vi "Navigation_no s curve may 2 encoders.vi"() -> ()   [LabVIEW 2015]
uses:
  <vilib>/myRIO/Instrument Drivers/Onboard IO/PWM/typedefs/PWM Reference.ctl
  <vilib>/myRIO/Common/Instrument Driver Framework/Utilities/typedefs/myRIO Generic Hardware Reference.ctl
  <vilib>/myRIO/Common/Instrument Driver Framework/Utilities/typedefs/Hardware Version Enum.ctl
  <vilib>/myRIO/Common/Instrument Driver Framework/Utilities/typedefs/myRIO v1.0 Reference.ctl
  <vilib>/myRIO/Common/Instrument Driver Framework/Utilities/typedefs/Generic FPGA Reference.ctl
  <vilib>/myRIO/Common/Instrument Driver Framework/myRIO v1.0/PWM/typedefs/PWM Channels Enum.ctl
  <vilib>/myRIO/Instrument Drivers/Onboard IO/PWM/typedefs/PWM Configuration.ctl
  <vilib>/userdefined/High Color/nirio_resource_hc.ctl
  <vilib>/myRIO/Common/Instrument Driver Framework/myRIO v1.0/PWM/vis/myRIO v1.1 Open PWM.vi
  <vilib>/myRIO/Common/Instrument Driver Framework/Utilities/vis/Validate Channels.vi
  <vilib>/myRIO/Common/Instrument Driver Framework/myRIO v1.0/PWM/vis/myRIO v1.0 Reserve PWM.vi
  <vilib>/myRIO/Common/Instrument Driver Framework/myRIO v1.0/PWM/vis/myRIO v1.0 Build MUX Configuration PWM.vi
  <vilib>/myRIO/Common/Instrument Driver Framework/myRIO v1.0/Resource Manager/vis/myRIO v1.0 Reserve Channel List.vi
  <vilib>/myRIO/Common/Instrument Driver Framework/myRIO v1.0/Resource Manager/vis/myRIO v1.0 Create Configuration List.vi
  <vilib>/myRIO/Common/Instrument Driver Framework/myRIO v1.0/Resource Manager/vis/myRIO v1.0 Reserve Channel.vi
  <vilib>/myRIO/Common/Instrument Driver Framework/myRIO v1.0/Resource Manager/vis/myRIO v1.0 Unreserve Channel.vi
  <vilib>/myRIO/Common/Instrument Driver Framework/myRIO v1.0/Resource Manager/vis/myRIO v1.0 Build Mutex Name.vi
  <vilib>/FPGAPlugInAG/myRIO-1900/niLvFpga_Open_myRIO-1900.vi
  <vilib>/rvi/interface/common/dynamic/niFpgaDynamicAddResources.vi
  <vilib>/myRIO/Common/Instrument Driver Framework/Utilities/vis/FPGA Ref Manager.vi
  <vilib>/Utility/error.llb/Error Cluster From Error Code.vi
  <vilib>/myRIO/Common/Instrument Driver Framework/Utilities/vis/Ref Counter.vi
  <vilib>/rvi/errors/niLvFpgaAdjustHostInterfaceError.vi
  <vilib>/Utility/VariantDataType/GetNumericInfo.vi
  <vilib>/myRIO/Common/Instrument Driver Framework/myRIO v1.0/myRIO v1.1 Open.vi
  <vilib>/myRIO/Common/Instrument Driver Framework/Utilities/vis/IO Manager.vi
  <vilib>/myRIO/Common/Instrument Driver Framework/Utilities/vis/Configuration Manager.vi
  <vilib>/myRIO/Common/Instrument Driver Framework/myRIO v1.0/Resource Manager/vis/myRIO v1.0 Configure IO.vi
  <vilib>/myRIO/Common/Instrument Driver Framework/myRIO v1.0/myRIO v1.0 Close.vi
  <vilib>/myRIO/Common/Instrument Driver Framework/myRIO v1.0/PWM/vis/myRIO v1.0 Write PWM.vi
  <vilib>/addons/control/pid/pid.llb/PID (DBL).vi
  <vilib>/rvi/interface/nirviOpenFPGA/nirviOpenFPGA.xnode
  FPGA Bitfiles/NavigationProjec_FPGATarget2_FPGAMainNavigati_PWPHW8gwDxI.lvbitx
  <vilib>/rvi/interface/nirviReadWriteControl/nirviReadWriteControl.xnode
  <vilib>/myRIO/Instrument Drivers/Onboard IO/PWM/vis/myRIO PWM Open.xnode
  <vilib>/myRIO/Instrument Drivers/Onboard IO/PWM/PWM.lvlib
  <vilib>/myRIO/Instrument Drivers/Utilities/Utilities.lvlib
  NiFpgaLv.dll
  <vilib>/rvi/interface/Simulation/niFpgaSimulationCallBeginRW.vi
  <vilib>/addons/control/pid/NI_PID_pid.lvlib
panel:
  out "percent to goal":dbl
  out "x goal current":dbl=8.0
  out "big red button":i16
  out "y1ahead":dbl
  out "angle error":dbl
  out "y desired":dbl
  out "slope desired":dbl
  out "orientation theta desired":dbl
  out "current angle":dbl
  out "current y":dbl
  out "current x":dbl
  out "mining angle":dbl
  out "mining y":dbl
  out "mining x":dbl
  out "mining location":dbl=1.0
  out "distance to goal":dbl
  out "loc_y":dbl
  out "loc_x":dbl
  out "loc_theta":dbl
  in  "motor killswitch":bool=TRUE
  in  "set start position":bool
  in  "dumping complete":bool
  in  "digging complete?":bool
  in  "position good?":bool
  in  "state":dbl
  in  "x goal":dbl=8.0
  in  "Encoder Reset":bool
  out "scale":dbl=1.0
  out "reset x y 2":dbl
  out "stop motors":dbl
  out "encoder stop switch":dbl=1.0
  out "left wheels actual pwm":dbl
  out "right wheels actual pwm":dbl
  out "desired pwm right":dbl
  out "desired pwm left":dbl
  out "left setpoint":dbl
  out "right setpoint":dbl
  in  "PID Settings":enum32{"Right PID PWM", "Left PID PWM"}(tab)
  in  "output range right":cluster{"output high":dbl, "output low":dbl}={"output high"=0.13333, "output low"=-0.13333} {"output low" format="%.6f"; "output high" format="%.5f"}
  in  "PID gains right":T1={"proportional gain (Kc)"=0.002, "integral time (Ti, min)"=7e-07, "derivative time (Td, min)"=0.0} {"derivative time (Td, min)" format="%.8f"; "integral time (Ti, min)" format="%.8f"; "proportional gain (Kc)" format="%.8f"}
  out "dt out (s) right":dbl format="%.3f"
  out "PID feedback Right":dbl
  out "Elapsed Time (s) Right":dbl caption="Elapsed Time (s)"
  in  "pid reset right":bool
  in  "output range left":cluster{"output high":dbl, "output low":dbl}={"output high"=0.13333, "output low"=-0.13333} {"output low" format="%.6f"; "output high" format="%.5f"}
  in  "PID gains left":T1={"proportional gain (Kc)"=0.002, "integral time (Ti, min)"=7e-07, "derivative time (Td, min)"=0.0} {"derivative time (Td, min)" format="%.8f"; "integral time (Ti, min)" format="%.8f"; "proportional gain (Kc)" format="%.8f"}
  out "dt out (s) left":dbl format="%.3f"
  out "PID feedback Left":dbl
  out "Elapsed Time (s) Left":dbl caption="Elapsed Time (s)"
  in  "pid reset left":bool
  out "start angle":dbl=1.0
  out "start x":dbl=1.0
  out "start y":dbl
  in  "stuff that i dont want to mess with right now":T2(tab)
  out "RM Linear Velocity (rot/s)":dbl
  out "RR Rot Velocity (rot/s)":dbl
  out "LR Rot Velocity (rot/s)":dbl
  out "LM Rot Velocity (rot/s)":dbl
  out "LF Rot Velocity (rot/s)":dbl
  out "RF Linear Velocity (rot/s)":dbl
  out "Tick Count(mSec) 2":u32 caption="Tick Count(mSec)"
  out "y traveled 2":dbl
  out "x traveled 2":dbl
  out "y position 2":dbl
  out "x position 2":dbl
  out "y dot 2":dbl
  out "distance traveled 2":dbl
  out "psi dot 2":dbl
  out "x dot 2":dbl
  out ".not. x? 2":bool
  out ".not. x? 3":bool
  out "goal reached":bool=TRUE
  out "avg ENC.B":dbl
  out "avg ENC.A":dbl
  out "ENC.B_c.CNTR":i32
  out "ENC.B_b.CNTR":i32
  out "ENC.B_a.CNTR":i32
  out "ENC.A_c.CNTR":i32
  out "ENC.A_b.CNTR":i32
  out "ENC.A_a.CNTR":i32
  out "stage set point parameters":T3(tab)
  in  "x straight 1 end":dbl=2.0
  in  "ypstart straight 1":dbl
  in  "ystart":dbl=1.0
  in  "yend straight 1":dbl=2.0
  in  "ypend straight 1":dbl
  out "a":dbl
  out "b":dbl
  out "c":dbl
  out "d":dbl
  out "x turn end":dbl=7.0
  out "x straight 2 end":dbl=10.0
  in  "mining y 1":dbl=2.0
  in  "mining angle 1":dbl
  in  "mining x 1":dbl=-8.0
  in  "mining angle -1":dbl
  in  "mining y -1":dbl=4.0
  in  "mining x -1":dbl=-8.0
  out "left pwm":dbl(graph)
  out "right pwm":dbl(graph)
  out "SYS.SELECTA":u8 format="%08b"
  in  "R Min Linear Velocity (ft/s)":dbl=-2.0 format="%#_13g"
  in  "R Max Linear Velocity (ft/s)":dbl=2.0 format="%#_13g"
  in  "L Min Linear Velocity (ft/s)":dbl=-2.0 format="%#_13g"
  in  "L Max Linear Velocity (ft/s)":dbl=2.0 format="%#_13g"
  out "Current Rot Velocity (rot/s)":T4(graph)
  # "Position Information"
  # "move cases along"
  # "end state 0\ngo to state 1"
  # "end state 1\ngo to state 2"
  # "end state 2\ngo to state 3"
  # "end state 3\ngo to state 4"
  # "end state 4\ngo to state 0"
  # "same thing, redundant \nbut can be changed to \nsomething useful later"
  # "this must be true to \ninitialize the routine"
  # "go through the 3\n movement cases"
  # "go through the 3\n movement cases"
  # "Stop Flags \n1=go \n0=stop"
  # "PWM Setpoint"
  # "Initial condtions"
  # "Encoder Values"
  # "Motor Control Parameters"
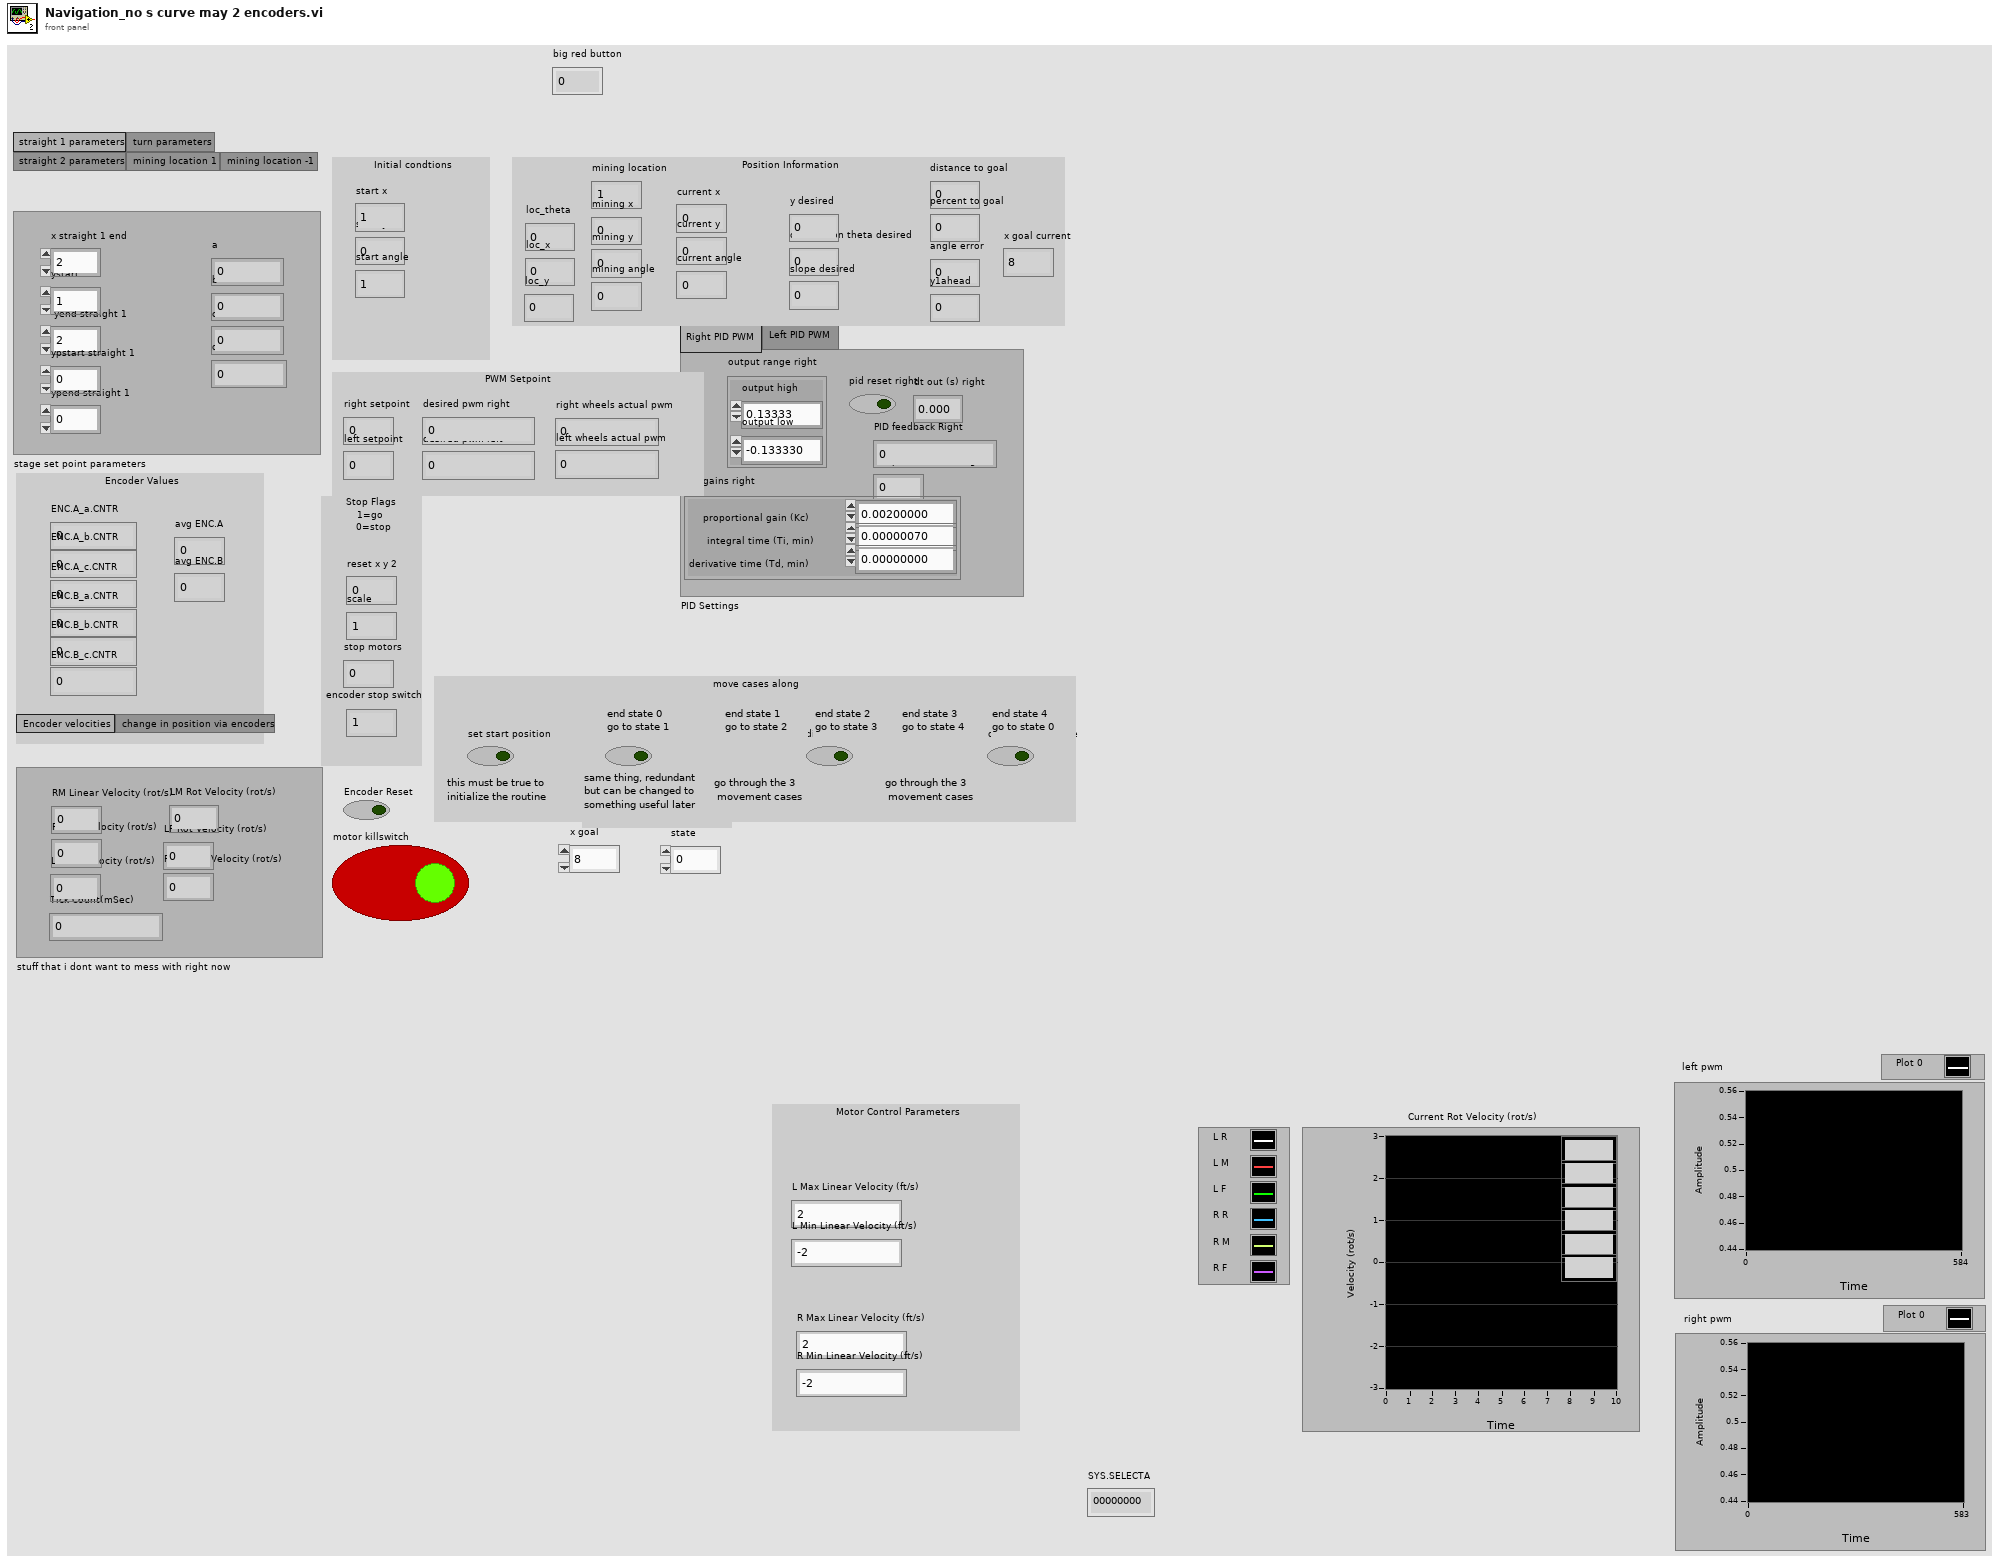
[diagram p1: front panel]
types:
  T1 = cluster{"proportional gain (Kc)":dbl, "integral time (Ti, min)":dbl, "derivative time (Td, min)":dbl}
  T2 = enum32{"Encoder velocities", "change in position via encoders"}
  T3 = enum32{"straight 1 parameters", "turn parameters", "straight 2 parameters", "mining location 1", "mining location -1"}
  T4 = cluster{"Rotational Velocity (RPS)":dbl, "Rotational Velocity (RPS)":dbl, "Rotational Velocity (RPS)":dbl, "Rotational Velocity (RPS)":dbl, "Rotational Velocity (RPS)":dbl, "Rotational Velocity (RPS)":dbl}
  T5 = typedef "nirio_resource_hc.ctl" = tag
  T6 = typedef "Hardware Version Enum.ctl" = enum16{"Unknown", "myRIO-1900", "myRIO-1950", "roboRIO"}
  T7 = typedef "PWM.lvlib/PWM Reference.ctl" = cluster{"myRIO Reference":T8, "PWM Channels Enum":T11, "PWM Configuration":T12}
  T8 = typedef "myRIO Generic Hardware Reference.ctl" = cluster{"myRIO Model":T6, "myRIO Hardware Reference":T9}
  T9 = typedef "myRIO v1.0 Reference.ctl" = cluster{"Generic FPGA Reference":T10, "Allow multiple opens":bool}
  T10 = typedef "Generic FPGA Reference.ctl" = refnum<k20>
  T11 = typedef "PWM Channels Enum.ctl" = enum16{"Not Connected", "C/PWM0", "C/PWM1", "A/PWM0", "A/PWM1", "A/PWM2", "B/PWM0", "B/PWM1", "B/PWM2", "PWM/PWM0", "PWM/PWM1", "PWM/PWM2", "PWM/PWM3", "PWM/PWM4", "PWM/PWM5", "PWM/PWM6", "PWM/PWM7", "PWM/PWM8", "PWM/PWM9"}
  T12 = typedef "PWM.lvlib/PWM Configuration.ctl" = cluster{"Frequency":dbl, "Duty Cycle":dbl}
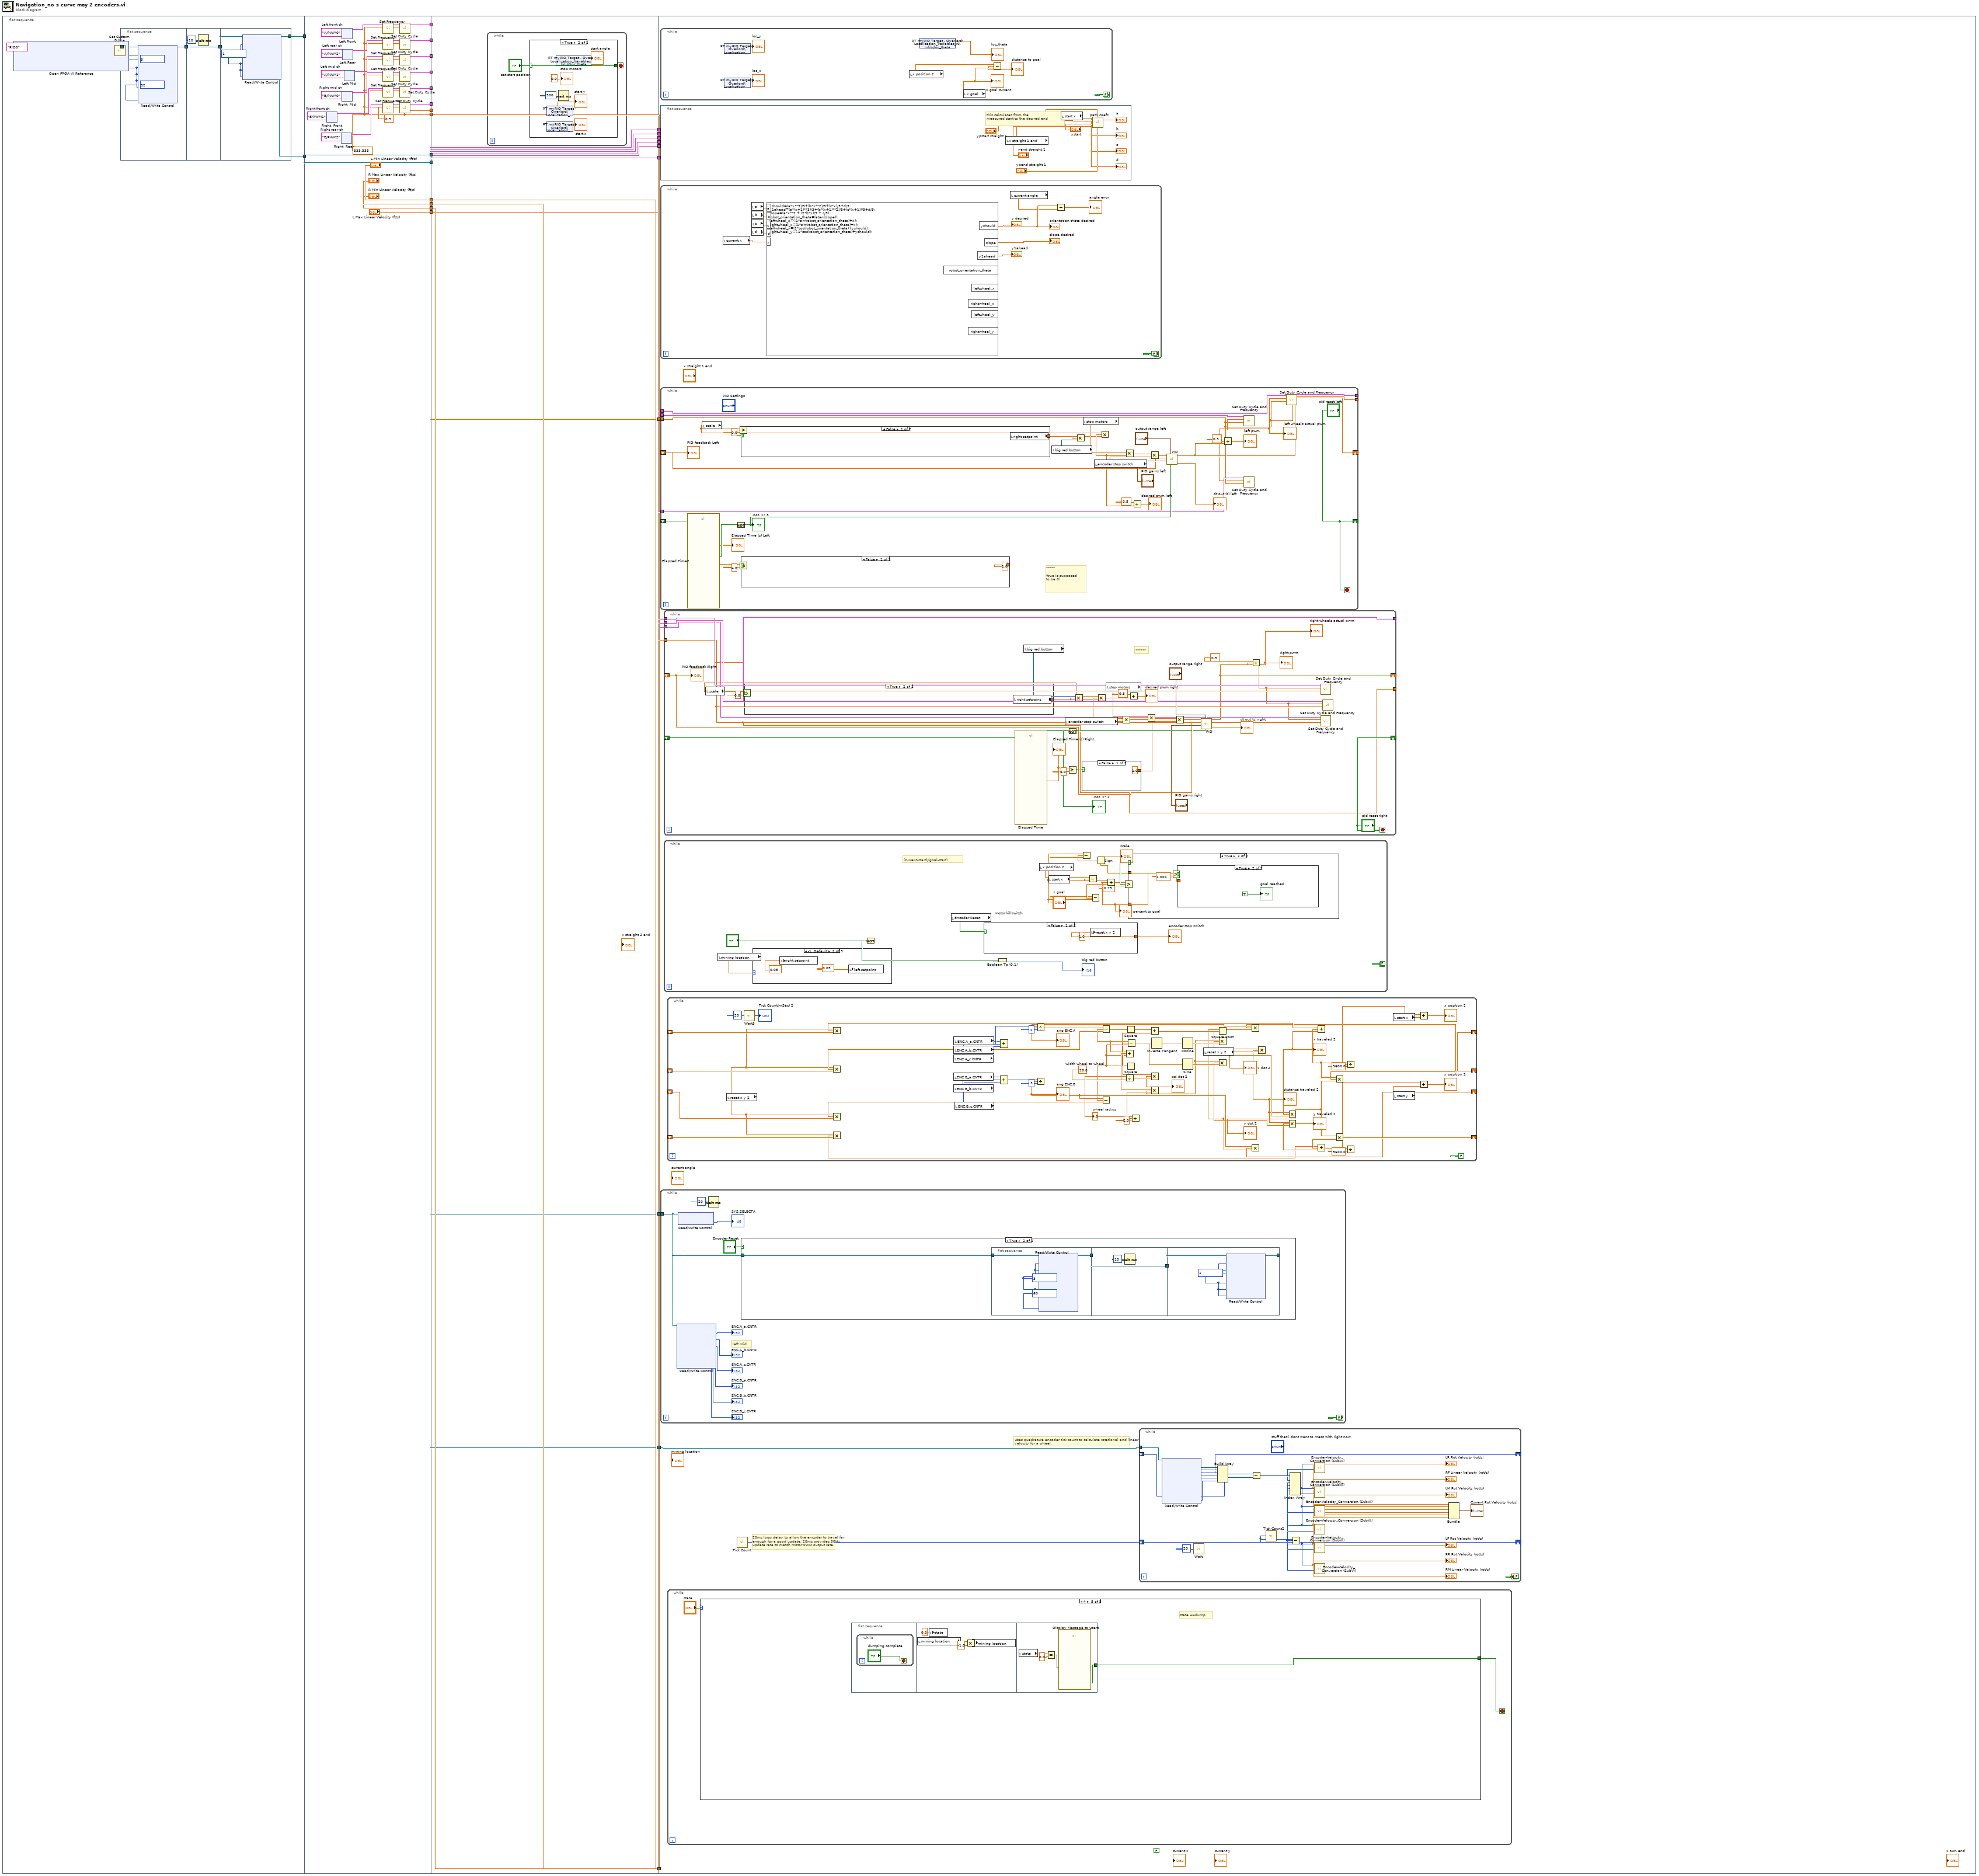
[diagram p0: block diagram]
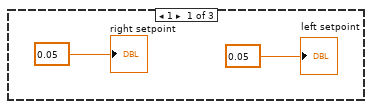
[diagram p3: hidden frame]
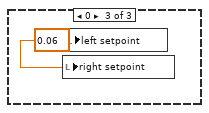
[diagram p4: hidden frame]
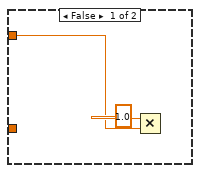
[diagram p5: hidden frame]
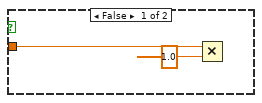
[diagram p6: hidden frame]
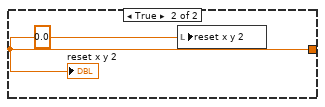
[diagram p7: hidden frame]
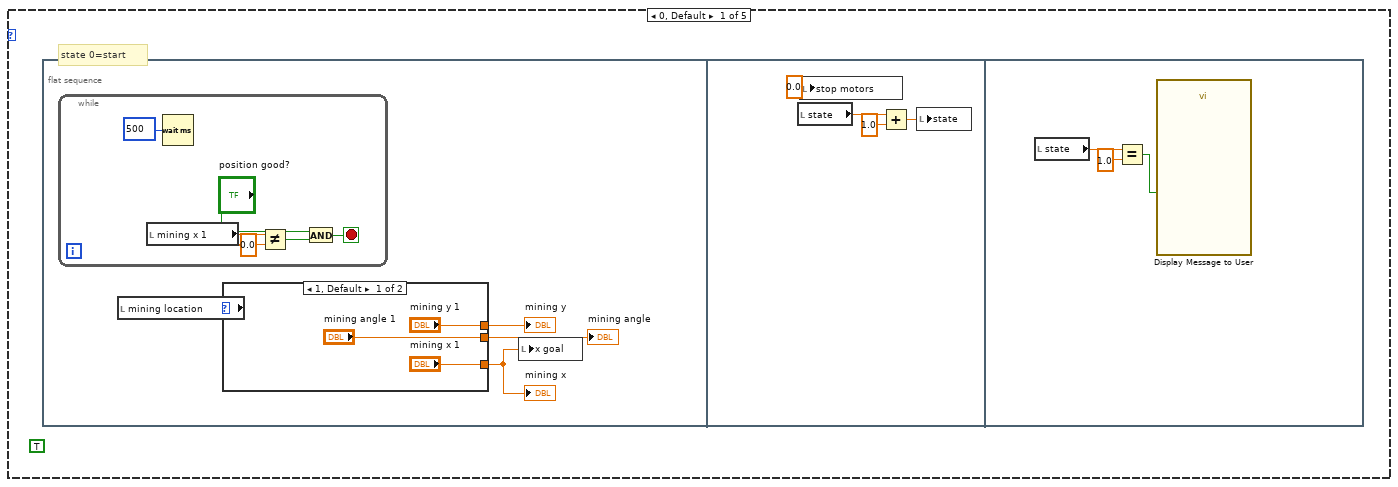
[diagram p8: hidden frame]
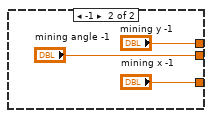
[diagram p9: hidden frame]
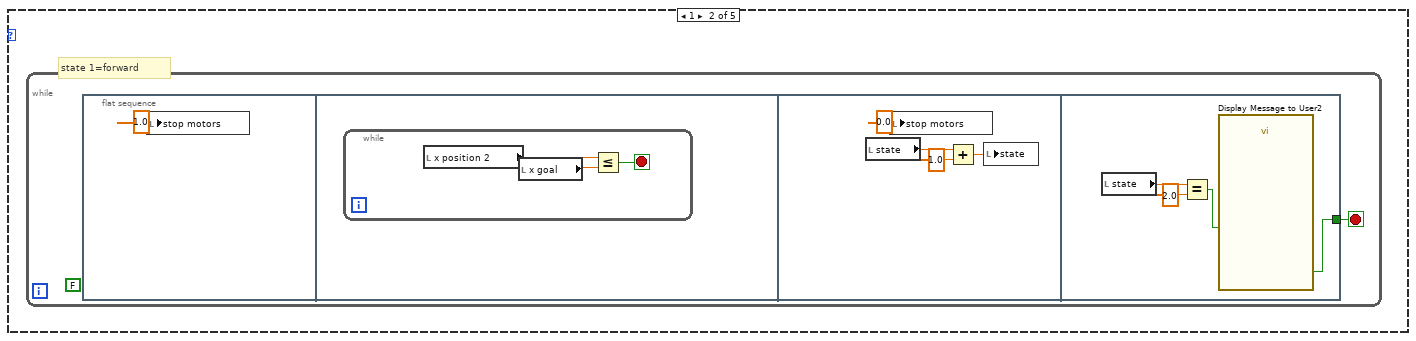
[diagram p10: hidden frame]
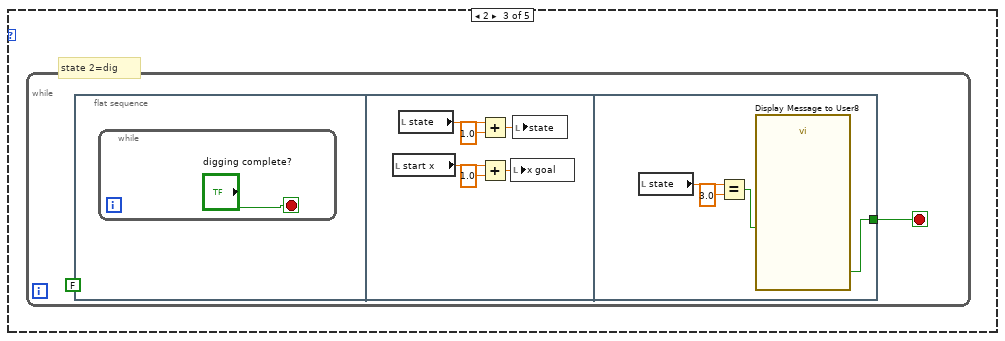
[diagram p11: hidden frame]
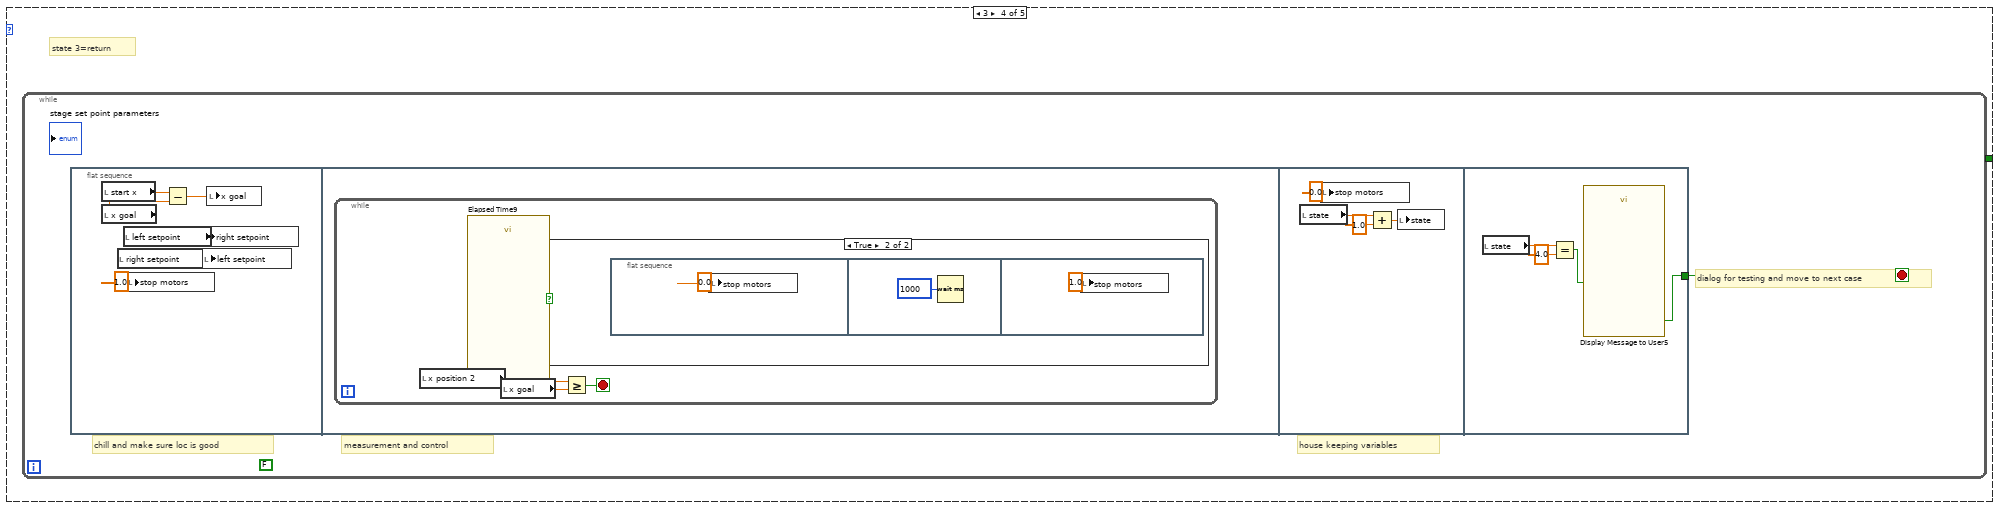
[diagram p12: hidden frame]
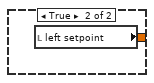
[diagram p14: hidden frame]
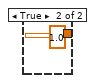
[diagram p15: hidden frame]
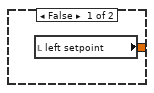
[diagram p16: hidden frame]
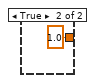
[diagram p17: hidden frame]
diagram:
  n1 = flat-sequence {
    tunnel: [w33] -> w30
    tunnel: [w33] -> w29
    tunnel: [w46] -> w28
    tunnel: [w61] -> w26
    tunnel: [w57] -> w24
    tunnel: [w56] -> w22
    tunnel: [w55] -> w20
    tunnel: [w54] -> w18
    tunnel: [w53] -> w16
    tunnel: ["L Max Linear Velocity (ft/s)"] -> w14
    tunnel: ["L Min Linear Velocity (ft/s)"] -> w12
    tunnel: ["R Max Linear Velocity (ft/s)"] -> w10
    tunnel: ["R Min Linear Velocity (ft/s)"] -> w8
    tunnel: [w48] -> w6
    tunnel: w30 -> [w47]
    tunnel: [w47] -> w4
    tunnel: w29 -> [w48]
    tunnel: [w46] -> w2
    tunnel: w28 -> [w187]
    tunnel: [w187] -> w27
    tunnel: w26 -> [w186]
    tunnel: [w186] -> w25
    tunnel: w24 -> [w185]
    tunnel: [w185] -> w23
    tunnel: w22 -> [w184]
    tunnel: [w184] -> w21
    tunnel: w20 -> [w183]
    tunnel: [w183] -> w19
    tunnel: w18 -> [w182]
    tunnel: [w182] -> w17
    tunnel: w16 -> [w181]
    tunnel: [w181] -> w15
    tunnel: w14 -> [w180]
    tunnel: [w180] -> w13
    tunnel: w12 -> [w179]
    tunnel: [w179] -> w11
    tunnel: w10 -> [w178]
    tunnel: [w178] -> w9
    tunnel: w8 -> [w177]
    tunnel: [w177] -> w7
    tunnel: w6 -> [w176]
    tunnel: [w176] -> w5
    tunnel: w4 -> [w175]
    tunnel: [w175] -> w3
    tunnel: w2 -> [w174]
    tunnel: [w174] -> w1
    tunnel: w27 -> [_]
    tunnel: w25 -> [w196]
    tunnel: w23 -> [w202]
    tunnel: w21 -> [w199]
    tunnel: w19 -> [w198]
    tunnel: w17 -> [w197]
    tunnel: w15 -> [w201]
    tunnel: w13 -> [_]
    tunnel: w11 -> [_]
    tunnel: w9 -> [_]
    tunnel: w7 -> [_]
    tunnel: w5 -> [w204]
    tunnel: w3 -> [w203]
    tunnel: w1 -> [w200]
    frame #0 {
      n2 = xnode "Open FPGA VI Reference"("resource name"=tag "RIO0") -> ("FPGA VI Reference Out"=w32:refnum<k20>)  [unwired: 1 in, 1 out]
      n3 = call <vilib>:"Set Custom Bitfile.vi"("Custom FPGA Reference In"=w32) -> ("Custom FPGA Reference Out"=w34:refnum<k20>)  [unwired: 9 in, 1 out]
      n4 = flat-sequence {
        tunnel: w34 -> [w39]
        tunnel: [w37] -> w36
        tunnel: w36 -> [w41]
        tunnel: [w41] -> w35
        tunnel: w35 -> [w44]
        tunnel: [w43] -> w33
        frame #0 {
          w38 = u8 32 ("SYS.SELECTA")
          w40 = u8 3 ("ENC.B_c.CNFG")
          n5 = xnode "Read/Write Control"("FPGA VI Reference In"=w39, "ENC.A_a.CNFG"=w40, "ENC.A_b.CNFG"=w40, "ENC.A_c.CNFG"=w40, "ENC.B_a.CNFG"=w40, "ENC.B_b.CNFG"=w40, "ENC.B_c.CNFG"=w40, "SYS.SELECTA"=w38, "SYS.SELECTB"=w38) -> ("FPGA VI Reference Out"=w37:refnum<k20>)  [unwired: 1 in, 1 out]
        }
        frame #1 {
          n6 = Wait (ms)(milliseconds to wait=u32 10) -> ()  [unwired: 1 out]
        }
        frame #2 {
          w45 = u8 1 ("ENC.B_c.CNFG")
          n7 = xnode "Read/Write Control"("FPGA VI Reference In"=w44, "ENC.A_a.CNFG"=w45, "ENC.A_b.CNFG"=w45, "ENC.A_c.CNFG"=w45, "ENC.B_a.CNFG"=w45, "ENC.B_b.CNFG"=w45, "ENC.B_c.CNFG"=w45) -> ("FPGA VI Reference Out"=w43:refnum<k20>)  [unwired: 1 in, 1 out]
        }
      }
    }
    frame #1 {
      w58 = 0.5 ("Duty Cycle")
      w46 = 333.333 ("Frequency [Hz]")
      w72 = tag "B/PWM2"  # Right rear ch
      w73 = tag "B/PWM0"  # Right mid ch
      w74 = tag "B/PWM1"  # Right front ch
      w75 = tag "A/PWM2"  # Left rear ch
      w76 = tag "A/PWM1"  # Left mid ch
      w77 = tag "A/PWM0"  # Left front ch
      n8 = xnode "Right  Front"("Channel Name"=w74) -> ("PWM Ref Out"=w68:T7)  [unwired: 2 in, 1 out]
      n9 = xnode "Right  Rear"("Channel Name"=w72) -> ("PWM Ref Out"=w66:T7)  [unwired: 2 in, 1 out]
      n10 = xnode "Left Front"("Channel Name"=w77) -> ("PWM Ref Out"=w71:T7)  [unwired: 2 in, 1 out]
      n11 = xnode "Right  Mid"("Channel Name"=w73) -> ("PWM Ref Out"=w67:T7)  [unwired: 2 in, 1 out]
      n12 = xnode "Left Rear"("Channel Name"=w75) -> ("PWM Ref Out"=w69:T7)  [unwired: 2 in, 1 out]
      n13 = xnode "Left Mid"("Channel Name"=w76) -> ("PWM Ref Out"=w70:T7)  [unwired: 2 in, 1 out]
      n14 = call <vilib>:"Set Frequency.vi"("Frequency [Hz]"=w46, "PWM Ref In"=w71) -> ("PWM Ref Out"=w65:T7)  [unwired: 7 in, 1 out]
      n15 = call <vilib>:"Set Frequency.vi"("Frequency [Hz]"=w46, "PWM Ref In"=w69) -> ("PWM Ref Out"=w60:T7)  [unwired: 7 in, 1 out]
      n16 = call <vilib>:"Set Frequency.vi"("Frequency [Hz]"=w46, "PWM Ref In"=w70) -> ("PWM Ref Out"=w59:T7)  [unwired: 7 in, 1 out]
      n17 = call <vilib>:"Set Frequency.vi"("Frequency [Hz]"=w46, "PWM Ref In"=w67) -> ("PWM Ref Out"=w63:T7)  [unwired: 7 in, 1 out]
      n18 = call <vilib>:"Set Frequency.vi"("Frequency [Hz]"=w46, "PWM Ref In"=w68) -> ("PWM Ref Out"=w62:T7)  [unwired: 7 in, 1 out]
      n19 = call <vilib>:"Set Frequency.vi"("Frequency [Hz]"=w46, "PWM Ref In"=w66) -> ("PWM Ref Out"=w64:T7)  [unwired: 7 in, 1 out]
      n20 = call <vilib>:"Set Duty Cycle.vi"("Duty Cycle"=w58, "PWM Ref In"=w65) -> ("PWM Ref Out"=w53:T7)  [unwired: 7 in, 1 out]
      n21 = call <vilib>:"Set Duty Cycle.vi"("Duty Cycle"=w58, "PWM Ref In"=w60) -> ("PWM Ref Out"=w61:T7)  [unwired: 7 in, 1 out]
      n22 = call <vilib>:"Set Duty Cycle.vi"("Duty Cycle"=w58, "PWM Ref In"=w59) -> ("PWM Ref Out"=w54:T7)  [unwired: 7 in, 1 out]
      n23 = call <vilib>:"Set Duty Cycle.vi"("Duty Cycle"=w58, "PWM Ref In"=w63) -> ("PWM Ref Out"=w56:T7)  [unwired: 7 in, 1 out]
      n24 = call <vilib>:"Set Duty Cycle.vi"("Duty Cycle"=w58, "PWM Ref In"=w62) -> ("PWM Ref Out"=w57:T7)  [unwired: 7 in, 1 out]
      n25 = call <vilib>:"Set Duty Cycle.vi"("Duty Cycle"=w58, "PWM Ref In"=w64) -> ("PWM Ref Out"=w55:T7)  [unwired: 7 in, 1 out]
    }
    frame #2 {
      n26 = while {
        stop <- w188 stop-if-true
        n27 = case shown="True" "set start position" {
          selector: "set start position" -> [_ w195]
          tunnel: [_ w195] -> w188
          frame False {
          }
          frame True {
            n28 = shared-variable "RT myRIO Target - Overlord\\Localization_Variables_r0.lvlib\\loc_y"() -> (→"start y":dbl)  [unwired: 1 in, 1 out]
            n29 = shared-variable "RT myRIO Target - Overlord\\Localization_Variables_r0.lvlib\\loc_x"() -> (→"start x":dbl)  [unwired: 1 in, 1 out]
            n30 = shared-variable "RT myRIO Target - Overlord\\Localization_Variables_r0.lvlib\\loc_theta"() -> (→"start angle":dbl)  [unwired: 1 in, 1 out]
            n31 = Wait (ms)(milliseconds to wait=u32 500) -> ()  [unwired: 1 out]
            "stop motors" <- 0.0 ("stop motors")
          }
        }
      }
    }
    frame #3 {
      (unwired) FALSE
      # "Uses quadrature encoder tick count to calculate rotational and linear velocity for a wheel."
      # "20ms loop delay to allow the encoder to travel far enough for a good update. 20ms provides 50Hz update rate to match motor PWM output rate."
      n32 = while {
        stop <- FALSE stop-if-true
        n33 = shared-variable "RT myRIO Target - Overlord\\Localization_Variables_r0.lvlib\\loc_y"() -> (→"loc_y":dbl)  [unwired: 1 in, 1 out]
        n34 = shared-variable "RT myRIO Target - Overlord\\Localization_Variables_r0.lvlib\\loc_x"() -> (→"loc_x":dbl)  [unwired: 1 in, 1 out]
        n35 = local read "x position 2"() -> (w343:dbl)
        n36 = shared-variable "RT myRIO Target - Overlord\\Localization_Variables_r0.lvlib\\loc_theta"() -> (→"loc_theta":dbl)  [unwired: 1 in, 1 out]
        n37 = local read "x goal"() -> (w346:dbl)
        "x goal current" <- w346
        n38 = Subtract(x=w343, y=w346) -> (x-y=→"distance to goal":dbl)
      }
      n39 = flat-sequence {
        frame #0 {
          # "this calculates from the \nmeasured start to the desired end"
          n40 = local read "x straight 1 end"() -> (w251:dbl)
          n41 = local read "start x"() -> (w252:dbl)
          n42 = call "path coefs.vi"("ypend"="ypend straight 1", "ypstart"="ypstart straight 1", "yend"="yend straight 1", "ystart"="ystart", "xend"=w251, "xstart"=w252) -> ("d"=→"d":dbl, "c"=→"c":dbl, "b"=→"b":dbl, "a"=→"a":dbl)  [unwired: 2 in]
        }
      }
      n43 = while {
        stop <- FALSE stop-if-true
        n44 = local read "current x"() -> (w245:dbl)
        n45 = local read "a"() -> (w249:dbl)
        n46 = local read "b"() -> (w248:dbl)
        n47 = local read "d"() -> (w246:dbl)
        n48 = local read "c"() -> (w247:dbl)
        n49 = formula code="yshould=(a*x**3)/3+(b*x**2)/3+(c*x)/3+d/3;\ny1ahead=(a*(x+1)**3)/3+(b*(x+1)**2)/3+(c*(x+1))/3+d/3;\nslope=(a*x**2 + (2*b*x)/3 + c/3);\nrobot_orientation_theta=(atan(slope));\nleftwheel_x=(-1*sin(robot_orientation_theta)+x);\nrightwheel_x=(1*sin(robot_orientation_theta)+x);\nleftwheel_y=(1*cos(robot_orientation_theta)+yshould);\nrightwheel_y=(-1*cos(robot_orientation_theta)+yshould);"("a"=w249, "b"=w248, "c"=w247, "d"=w246, "x"=w245) -> ("yshould"=→"y desired":dbl, "slope"=→"slope desired":dbl, "robot_orientation_theta"=w242:dbl, "y1ahead"=→"y1ahead":dbl)  [unwired: 4 out]
        "orientation theta desired" <- w242
        n50 = local read "current angle"() -> (w241:dbl)
        n51 = Subtract(x=w242, y=w241) -> (x-y=→"angle error":dbl)
      }
      n52 = while {
        tunnel: w201 -> [w380]
        tunnel: [w381] -> _
        tunnel: w200 -> [w368]
        shift-right: [w367] -> _
        shift-left: _ -> [w376]
        shift-right: ["pid reset left"] -> _
        shift-left: _ -> [w362]
        tunnel: [w368] -> _
        tunnel: w197 -> [w370]
        tunnel: w196 -> [w369]
        stop <- "pid reset left" stop-if-true
        # "*****\n\n(true is supposed\nto be 0)"
        n53 = call "Elapsed Time2"("Reset"=w362) -> ("Elapsed Time (s)"=w361:dbl, "Time has Elapsed"=w363:bool)  [unwired: 11 in, 6 out]
        "Elapsed Time (s) Left" <- w361
        n54 = local read "scale"() -> (w353:dbl)
        n55 = Not(x=w363) -> (.not. x?=w375:bool)
        ".not. x? 3" <- w375
        n56 = Greater?(x=w353, y=0.0) -> (0:w356:bool)
        n57 = Greater Or Equal?(x=w361, y=4.0) -> (x >= y?=w359:bool)
        n58 = case shown="False" w356 {
          tunnel: [w382 w383] -> w366
          frame False {
            n59 = local read "right setpoint"() -> (w382:dbl)
          }
          frame True {
            n60 = local read "left setpoint"() -> (w383:dbl)
          }
        }
        n61 = case shown="False" w359 {
          tunnel: [1.0 1.0] -> _
          frame False {
          }
          frame True {
          }
        }
        n62 = local read "big red button"() -> (w350:i16)
        n63 = Multiply(x=w366, y=w350) -> (x*y=w351:dbl)
        n64 = local read "stop motors"() -> (w371:dbl)
        n65 = local read "encoder stop switch"() -> (w364:dbl)
        n66 = Multiply(x=w353, y=w351) -> (x*y=w354:dbl)
        n67 = Multiply(x=w371, y=w354) -> (x*y=w365:dbl)
        n68 = Add(x=0.5, y=w354) -> (x+y=→"desired pwm left":dbl)
        n69 = Multiply(x=w365, y=w364) -> (x*y=w352:dbl)
        n70 = call-poly <vilib>:"PID.vi"("reinitialize? (F)"=w375, "output range"="output range left", "PID gains"="PID gains left", "process variable"=w376, "setpoint"=w352) -> ("dt out (s)"=→"dt out (s) left":dbl, "output"=w367:dbl)  [unwired: 5 in]
        n71 = Add(x=0.5, y=w367) -> (x+y=w357:dbl)
        "left wheels actual pwm" <- w357
        "left pwm" <- w357
        n72 = call <vilib>:"Set Duty Cycle and Frequency.vi"("Frequency [Hz]"=w368, "Duty Cycle"=w357, "PWM Ref In"=w369) -> ()  [unwired: 6 in, 2 out]
        n73 = call <vilib>:"Set Duty Cycle and Frequency.vi"("Frequency [Hz]"=w368, "Duty Cycle"=w357, "PWM Ref In"=w370) -> ()  [unwired: 6 in, 2 out]
        n74 = call <vilib>:"Set Duty Cycle and Frequency.vi"("Frequency [Hz]"=w368, "Duty Cycle"=w357, "PWM Ref In"=w380) -> ("PWM Ref Out"=w381:T7)  [unwired: 6 in, 1 out]
        "PID feedback Left" <- w376
      }
      n75 = while {
        tunnel: w204 -> [w486]
        stop <- FALSE stop-if-true
        # "left mid"
        n76 = xnode "Read/Write Control"("FPGA VI Reference In"=w486) -> ("ENC.A_a.CNTR"=→"ENC.A_a.CNTR":u32, "ENC.A_b.CNTR"=→"ENC.A_b.CNTR":u32, "ENC.A_c.CNTR"=→"ENC.A_c.CNTR":u32, "ENC.B_a.CNTR"=→"ENC.B_a.CNTR":u32, "ENC.B_b.CNTR"=→"ENC.B_b.CNTR":u32, "ENC.B_c.CNTR"=→"ENC.B_c.CNTR":u32)  [unwired: 1 in, 2 out]
        n77 = xnode "Read/Write Control"("FPGA VI Reference In"=w486) -> ("SYS.SELECTA"=→"SYS.SELECTA":u8)  [unwired: 1 in, 2 out]
        n78 = Wait (ms)(milliseconds to wait=u32 20) -> ()  [unwired: 1 out]
        n79 = case shown="True" "Encoder Reset" {
          tunnel: w486 -> [_ w497]
          frame False {
          }
          frame True {
            n80 = flat-sequence {
              tunnel: w497 -> [w502]
              tunnel: [w500] -> w499
              tunnel: w499 -> [w504]
              tunnel: [w504] -> w498
              tunnel: w498 -> [w507]
              tunnel: [w506] -> _
              frame #0 {
                w501 = u8 60 ("SYS.SELECTA")
                w503 = u8 3 ("ENC.B_c.CNFG")
                n81 = xnode "Read/Write Control"("FPGA VI Reference In"=w502, "ENC.A_a.CNFG"=w503, "ENC.A_b.CNFG"=w503, "ENC.A_c.CNFG"=w503, "ENC.B_a.CNFG"=w503, "ENC.B_b.CNFG"=w503, "ENC.B_c.CNFG"=w503, "SYS.SELECTA"=w501, "SYS.SELECTB"=w501) -> ("FPGA VI Reference Out"=w500:refnum<k20>)  [unwired: 1 in, 1 out]
              }
              frame #1 {
                n82 = Wait (ms)(milliseconds to wait=u32 10) -> ()  [unwired: 1 out]
              }
              frame #2 {
                w508 = u8 1 ("ENC.B_c.CNFG")
                n83 = xnode "Read/Write Control"("FPGA VI Reference In"=w507, "ENC.A_a.CNFG"=w508, "ENC.A_b.CNFG"=w508, "ENC.A_c.CNFG"=w508, "ENC.B_a.CNFG"=w508, "ENC.B_b.CNFG"=w508, "ENC.B_c.CNFG"=w508) -> ("FPGA VI Reference Out"=w506:refnum<k20>)  [unwired: 1 in, 1 out]
              }
            }
          }
        }
      }
      n84 = while {
        tunnel: w202 -> [w480]
        tunnel: [w481] -> _
        tunnel: [w469] -> _
        shift-right: [w468] -> _
        shift-left: _ -> [w476]
        shift-right: ["pid reset right"] -> _
        shift-left: _ -> [w462]
        tunnel: w200 -> [w469]
        tunnel: w199 -> [w471]
        tunnel: w198 -> [w470]
        stop <- "pid reset right" stop-if-true
        # "******"
        n85 = local read "scale"() -> (w455:dbl)
        n86 = Greater?(x=w455, y=0.0) -> (0:w453:bool)
        n87 = case shown="True" w453 {
          tunnel: [w482 w483] -> w452
          frame False {
            n88 = local read "left setpoint"() -> (w482:dbl)
          }
          frame True {
            n89 = local read "right setpoint"() -> (w483:dbl)
          }
        }
        n90 = call "Elapsed Time"("Reset"=w462) -> ("Elapsed Time (s)"=w461:dbl, "Time has Elapsed"=w459:bool)  [unwired: 11 in, 6 out]
        "Elapsed Time (s) Right" <- w461
        n91 = local read "big red button"() -> (w448:i16)
        n92 = local read "encoder stop switch"() -> (w465:dbl)
        n93 = Not(x=w459) -> (.not. x?=w475:bool)
        ".not. x? 2" <- w475
        n94 = Greater Or Equal?(x=w461, y=4.0) -> (x >= y?=w458:bool)
        n95 = Multiply(x=w448, y=w452) -> (x*y=w449:dbl)
        n96 = case shown="False" w458 {
          tunnel: [1.0 1.0] -> w463
          frame False {
          }
          frame True {
          }
        }
        n97 = Multiply(x=w455, y=w449) -> (x*y=w467:dbl)
        n98 = local read "stop motors"() -> (w456:dbl)
        n99 = Multiply(x=w467, y=w465) -> (x*y=w466:dbl)
        n100 = Add(x=0.5, y=w467) -> (x+y=→"desired pwm right":dbl)
        n101 = Multiply(x=w456, y=w466) -> (x*y=w457:dbl)
        n102 = Multiply(x=w457, y=w463) -> (x*y=w464:dbl)
        n103 = call-poly <vilib>:"PID.vi"("reinitialize? (F)"=w475, "output range"="output range right", "PID gains"="PID gains right", "process variable"=w476, "setpoint"=w464) -> ("dt out (s)"=→"dt out (s) right":dbl, "output"=w468:dbl)  [unwired: 5 in]
        n104 = Add(x=0.5, y=w468) -> (x+y=w450:dbl)
        "right wheels actual pwm" <- w450
        "right pwm" <- w450
        n105 = call <vilib>:"Set Duty Cycle and Frequency.vi"("Frequency [Hz]"=w469, "Duty Cycle"=w450, "PWM Ref In"=w471) -> ()  [unwired: 6 in, 2 out]
        n106 = call <vilib>:"Set Duty Cycle and Frequency.vi"("Frequency [Hz]"=w469, "Duty Cycle"=w450, "PWM Ref In"=w470) -> ()  [unwired: 6 in, 2 out]
        n107 = call <vilib>:"Set Duty Cycle and Frequency.vi"("Frequency [Hz]"=w469, "Duty Cycle"=w450, "PWM Ref In"=w480) -> ("PWM Ref Out"=w481:T7)  [unwired: 6 in, 1 out]
        "PID feedback Right" <- w476
      }
      n108 = while {
        stop <- FALSE stop-if-true
        # "(current-start)/(goal-start)"
        n109 = local read "mining location"() -> (w216:dbl)
        n110 = case shown="-1, Default" w216 {
          frame 1 {
            "right setpoint" <- 0.05
            "left setpoint" <- 0.05
          }
          frame -1, Default {
            n111 = local write "right setpoint"(0.05) -> ()
            n112 = local write "left setpoint"(0.05) -> ()
          }
          frame 0 {
            w227 = 0.06 ("left setpoint")
            n113 = local write "right setpoint"(w227) -> ()
            n114 = local write "left setpoint"(w227) -> ()
          }
        }
        n115 = Not(x="motor killswitch") -> (.not. x?=w220:bool)
        n116 = local read "Encoder Reset"() -> (w222:bool)
        n117 = case shown="False" w222 {
          tunnel: [w237 w238] -> w221
          frame False {
            w237 = 1.0
            n118 = local write "reset x y 2"(w237) -> ()
          }
          frame True {
            w238 = 0.0
            n119 = local write "reset x y 2"(w238) -> ()
            "reset x y 2" <- w238
          }
        }
        "encoder stop switch" <- w221
        n120 = Boolean To (0,1)(Boolean=w220) -> (0, 1=→"big red button":i16)
        n121 = local read "x position 2"() -> (w215:dbl)
        n122 = local read "start x"() -> (w211:dbl)
        n123 = Subtract(x="x goal", y=w211) -> (x-y=w210:dbl)
        n124 = Subtract(x=w215, y=w211) -> (x-y=w214:dbl)
        n125 = Subtract(x=w211, y="x goal") -> (x-y=w213:dbl)
        n126 = Sign(1:w210) -> (0:w206:dbl)
        "scale" <- w206
        n127 = Divide(x=w214, y=w213) -> (x/y=w207:dbl)
        "percent to goal" <- w207
        n128 = Greater?(x=w207, y=0.75) -> (0:w208:bool)
        n129 = case shown="True" w208 {
          tunnel: w206 -> [w228 w230]
          tunnel: w207 -> [_ w231]
          frame False {
            n130 = Multiply(x=1.0, y=w228) -> ()  [unwired: 1 out]
          }
          frame True {
            n131 = Greater?(x=w231, y=1.001) -> (0:w232:bool)
            n132 = case shown="True" w232 {
              tunnel: w230 -> [w235 _]
              frame False {
                n133 = Multiply(x=w235, y=1.0) -> ()  [unwired: 1 out]
              }
              frame True {
                "goal reached" <- TRUE
              }
            }
          }
        }
      }
      n134 = while {
        shift-right: [w396] -> _
        shift-left: _ -> [w434]
        shift-right: [w393] -> _
        shift-left: _ -> [w433]
        shift-right: [w395] -> _
        shift-left: _ -> [w408]
        shift-right: [w394] -> _
        shift-left: _ -> [w407]
        stop <- FALSE stop-if-true
        w429 = 28.0  # width wheel to wheel
        w430 = 4.0  # wheel radius
        n135 = local read "reset x y 2"() -> (w392:dbl)
        n136 = call "Wait3"("Count(mSec)"=u32 20) -> ("Tick Count(mSec)"=→"Tick Count(mSec) 2":u32)
        n137 = Multiply(x=w392, y=w407) -> (x*y=w398:dbl)
        n138 = Multiply(x=w392, y=w434) -> (x*y=w400:dbl)
        n139 = Multiply(x=w392, y=w433) -> (x*y=w397:dbl)
        n140 = Multiply(x=w392, y=w408) -> (x*y=w399:dbl)
        n141 = local read "ENC.A_b.CNTR"() -> (w441:i32)
        n142 = local read "ENC.A_c.CNTR"() -> (w440:i32)
        n143 = local read "ENC.B_a.CNTR"() -> (w439:i32)
        n144 = local read "ENC.B_b.CNTR"() -> (w438:i32)
        n145 = local read "ENC.A_a.CNTR"() -> (w442:i32)
        n146 = local read "ENC.B_c.CNTR"() -> (w437:i32)
        n147 = Compound Arithmetic op=ADD(w442, w441, w440) -> (w446:i32)
        n148 = Compound Arithmetic op=ADD(w439, w438, w437) -> (w445:i32)
        n149 = Divide(x=w446, y=2) -> (x/y=w435:dbl)
        "avg ENC.A" <- w435
        n150 = Divide(x=w445, y=3) -> (x/y=w432:dbl)
        "avg ENC.B" <- w432
        n151 = Subtract(x=w435, y=w400) -> (x-y=w423:dbl)
        n152 = Subtract(x=w432, y=w397) -> (x-y=w422:dbl)
        n153 = Add(x=w423, y=w422) -> (x+y=w427:dbl)
        n154 = Divide(x=w430, y=w429) -> (x/y=w425:dbl)
        n155 = Square(x=w423) -> (x^2=w420:dbl)
        n156 = Square(x=w422) -> (x^2=w421:dbl)
        n157 = Subtract(x=w423, y=w422) -> (x-y=w426:dbl)
        n158 = Divide(x=w430, y=2.0) -> (x/y=w428:dbl)
        n159 = Add(x=w420, y=w421) -> (x+y=w419:dbl)
        n160 = Multiply(x=w426, y=w425) -> (x*y=→"psi dot 2":dbl)
        n161 = Multiply(x=w427, y=w428) -> (x*y=w416:dbl)
        n162 = Inverse Tangent(1:w426) -> (0:w424:dbl)
        n163 = Cosine(x=w424) -> (cos(x)=w417:dbl)
        n164 = Sine(x=w424) -> (sin(x)=w418:dbl)
        n165 = local read "reset x y 2"() -> (w390:dbl)
        n166 = Square Root(x=w419) -> (sqrt(x)=w413:dbl)
        n167 = Multiply(x=w416, y=w417) -> (x*y=w414:dbl)
        "x dot 2" <- w414
        n168 = Multiply(x=w416, y=w418) -> (x*y=w415:dbl)
        "y dot 2" <- w415
        n169 = Multiply(x=w435, y=w390) -> (x*y=w396:dbl)
        n170 = Multiply(x=w432, y=w390) -> (x*y=w393:dbl)
        n171 = Multiply(x=w413, y=w390) -> (x*y=w391:dbl)
        "distance traveled 2" <- w391
        n172 = Multiply(x=w391, y=w414) -> (x*y=w412:dbl)
        "x traveled 2" <- w412
        n173 = Multiply(x=w391, y=w415) -> (x*y=w411:dbl)
        "y traveled 2" <- w411
        n174 = Add(x=w398, y=w412) -> (x+y=w410:dbl)
        n175 = Add(x=w399, y=w411) -> (x+y=w402:dbl)
        n176 = Multiply(x=w410, y=w390) -> (x*y=w394:dbl)
        n177 = Multiply(x=w390, y=w402) -> (x*y=w395:dbl)
        n178 = Divide(x=w410, y=9600.0) -> (x/y=w405:dbl)
        n179 = Divide(x=w402, y=9600.0) -> (x/y=w406:dbl)
        n180 = local read "start x"() -> (w403:dbl)
        n181 = local read "start y"() -> (w404:dbl)
        n182 = Add(x=w405, y=w403) -> (x+y=→"x position 2":dbl)
        n183 = Add(x=w406, y=w404) -> (x+y=→"y position 2":dbl)
      }
      n184 = while {
        stop <- w262 stop-if-true
        n185 = case shown="4" "state" {
          tunnel: [_ _ _ _ w333] -> w262
          frame 0, Default {
            (unwired) TRUE
            # "state 0=start"
            n186 = flat-sequence {
              frame #0 {
                n187 = while {
                  stop <- w273 stop-if-true
                  n188 = local read "mining x 1"() -> (w278:dbl)
                  n189 = Wait (ms)(milliseconds to wait=u32 500) -> ()  [unwired: 1 out]
                  n190 = Not Equal?(x=w278, y=0.0) -> (x != y?=w274:bool)
                  n191 = And(x="position good?", y=w274) -> (x .and. y?=w273:bool)
                }
                n192 = local read "mining location"() -> (w266:dbl)
                n193 = case shown="1, Default" w266 {
                  tunnel: ["mining x 1" "mining x -1"] -> w263
                  tunnel: ["mining y 1" "mining y -1"] -> w265
                  tunnel: ["mining angle 1" "mining angle -1"] -> w264
                  frame 1, Default {
                  }
                  frame -1 {
                  }
                }
                "mining x" <- w263
                "mining y" <- w265
                "mining angle" <- w264
                n194 = local write "x goal"(w263) -> ()
              }
              frame #1 {
                n195 = local read "state"() -> (w280:dbl)
                n196 = local write "stop motors"(0.0 ("stop motors")) -> ()
                n197 = Add(x=w280, y=1.0) -> (x+y=w282:dbl)
                n198 = local write "state"(w282) -> ()
              }
              frame #2 {
                n199 = local read "state"() -> (w285:dbl)
                n200 = Equal?(x=w285, y=1.0) -> (x = y?=w283:bool)
                n201 = call "Display Message to User"("Enable"=w283) -> ()  [unwired: 9 in, 2 out]
              }
            }
          }
          frame 1 {
            # "state 1=forward"
            n202 = while {
              stop <- w286 stop-if-true
              (unwired) FALSE
              n203 = flat-sequence {
                tunnel: [w295] -> w286
                frame #0 {
                  n204 = local write "stop motors"(1.0) -> ()
                }
                frame #1 {
                  n205 = while {
                    stop <- w290 stop-if-true
                    n206 = local read "x position 2"() -> (w288:dbl)
                    n207 = local read "x goal"() -> (w289:dbl)
                    n208 = Less Or Equal?(x=w288, y=w289) -> (x <= y?=w290:bool)
                  }
                }
                frame #2 {
                  n209 = local read "state"() -> (w291:dbl)
                  n210 = local write "stop motors"(0.0) -> ()
                  n211 = Add(x=w291, y=1.0) -> (x+y=w293:dbl)
                  n212 = local write "state"(w293) -> ()
                }
                frame #3 {
                  n213 = local read "state"() -> (w298:dbl)
                  n214 = Equal?(x=w298, y=2.0) -> (x = y?=w296:bool)
                  n215 = call "Display Message to User2"("Enable"=w296) -> ("OK"=w295:bool)  [unwired: 9 in, 1 out]
                }
              }
            }
          }
          frame 2 {
            # "state 2=dig"
            n216 = while {
              stop <- w299 stop-if-true
              (unwired) FALSE
              n217 = flat-sequence {
                tunnel: [w307] -> w299
                frame #0 {
                  n218 = while {
                    stop <- "digging complete?" stop-if-true
                  }
                }
                frame #1 {
                  n219 = local read "start x"() -> (w303:dbl)
                  n220 = local read "state"() -> (w305:dbl)
                  n221 = Add(x=w305, y=1.0) -> (x+y=w304:dbl)
                  n222 = Add(x=w303, y=1.0) -> (x+y=w302:dbl)
                  n223 = local write "x goal"(w302) -> ()
                  n224 = local write "state"(w304) -> ()
                }
                frame #2 {
                  n225 = local read "state"() -> (w310:dbl)
                  n226 = Equal?(x=w310, y=3.0) -> (x = y?=w308:bool)
                  n227 = call "Display Message to User8"("Enable"=w308) -> ("OK"=w307:bool)  [unwired: 9 in, 1 out]
                }
              }
            }
          }
          frame 3 {
            # "state 3=return"
            n228 = while {
              stop <- w311 stop-if-true
              (unwired) FALSE
              # "dialog for testing and move to next case"
              # "measurement and control"
              # "chill and make sure loc is good"
              # "house keeping variables"
              n229 = flat-sequence {
                tunnel: [w329] -> w311
                frame #0 {
                  n230 = local read "start x"() -> (w314:dbl)
                  n231 = local read "x goal"() -> (w312:dbl)
                  n232 = local read "right setpoint"() -> (w315:dbl)
                  n233 = local read "left setpoint"() -> (w316:dbl)
                  n234 = local write "stop motors"(1.0) -> ()
                  n235 = Subtract(x=w314, y=w312) -> (x-y=w313:dbl)
                  n236 = local write "right setpoint"(w316) -> ()
                  n237 = local write "left setpoint"(w315) -> ()
                  n238 = local write "x goal"(w313) -> ()
                }
                frame #1 {
                  n239 = while {
                    stop <- w321 stop-if-true
                    n240 = local read "x position 2"() -> (w318:dbl)
                    n241 = call "Elapsed Time9"() -> ("Time has Elapsed"=w320:bool)  [unwired: 12 in, 7 out]
                    n242 = local read "x goal"() -> (w319:dbl)
                    n243 = case shown="True" w320 {
                      frame False {
                      }
                      frame True {
                        n244 = flat-sequence {
                          frame #0 {
                            n245 = local write "stop motors"(0.0) -> ()
                          }
                          frame #1 {
                            n246 = Wait (ms)(milliseconds to wait=u32 1000) -> ()  [unwired: 1 out]
                          }
                          frame #2 {
                            n247 = local write "stop motors"(1.0) -> ()
                          }
                        }
                      }
                    }
                    n248 = Greater Or Equal?(x=w318, y=w319) -> (x >= y?=w321:bool)
                  }
                }
                frame #2 {
                  n249 = local read "state"() -> (w326:dbl)
                  n250 = local write "stop motors"(0.0) -> ()
                  n251 = Add(x=w326, y=1.0) -> (x+y=w328:dbl)
                  n252 = local write "state"(w328) -> ()
                }
                frame #3 {
                  n253 = local read "state"() -> (w332:dbl)
                  n254 = Equal?(x=w332, y=4.0) -> (x = y?=w330:bool)
                  n255 = call "Display Message to User5"("Enable"=w330) -> ("OK"=w329:bool)  [unwired: 9 in, 1 out]
                }
              }
            }
          }
          frame 4 {
            # "state 4=dump"
            n256 = flat-sequence {
              tunnel: [w339] -> w333
              frame #0 {
                n257 = while {
                  stop <- "dumping complete" stop-if-true
                }
              }
              frame #1 {
                n258 = local read "mining location"() -> (w337:dbl)
                n259 = local write "state"(0.0) -> ()
                n260 = Multiply(x=w337, y=-1.0) -> (x*y=w335:dbl)
                n261 = local write "mining location"(w335) -> ()
              }
              frame #2 {
                n262 = local read "state"() -> (w342:dbl)
                n263 = Equal?(x=w342, y=0.0) -> (x = y?=w340:bool)
                n264 = call "Display Message to User9"("Enable"=w340) -> ("OK"=w339:bool)  [unwired: 9 in, 1 out]
              }
            }
          }
        }
      }
      n265 = call "Tick Count"() -> ("Tick Count(uSec)"=w205:u32)
      n266 = while {
        shift-right: [w527] -> _
        shift-left: _ -> [w526]
        shift-right: [w524] -> _
        shift-left: w205 -> [w523]
        tunnel: w203 -> [w534]
        stop <- FALSE stop-if-true
        n267 = xnode "Read/Write Control"("FPGA VI Reference In"=w534) -> ("ENC.A_a.CNTR"=w533:u32, "ENC.A_b.CNTR"=w532:u32, "ENC.A_c.CNTR"=w531:u32, "ENC.B_a.CNTR"=w530:u32, "ENC.B_b.CNTR"=w529:u32, "ENC.B_c.CNTR"=w528:u32)  [unwired: 1 in, 2 out]
        n268 = call "Wait"("Count(mSec)"=u32 20) -> ()  [unwired: 1 out]
        n269 = Build Array(w533, w532, w531, w530, w529, w528) -> (w527:u32[])
        n270 = Subtract(x=w527, y=w526) -> (x-y=w525:u32[])
        n271 = call "Tick Count2"() -> ("Tick Count(uSec)"=w524:u32)
        n272 = Index Array(array=w525) -> (element #1=w522:u32, element #2=w521:u32, element #3=w520:u32, element #4=w519:u32, element #5=w518:u32, element #6=w517:u32)  [unwired: 6 in]
        n273 = Subtract(x=w524, y=w523) -> (x-y=w516:u32)
        n274 = call "Encoder-Velocity_Conversion (SubVI).vi"("delta  Encoder Count"=w522, "dt (uSec)"=w516) -> ("Rotational Velocity (RPS)"=w512:dbl)  [unwired: 7 in, 2 out]
        "LR Rot Velocity (rot/s)" <- w512
        n275 = call "Encoder-Velocity_Conversion (SubVI).vi"("delta  Encoder Count"=w517, "dt (uSec)"=w516) -> ("Rotational Velocity (RPS)"=w514:dbl)  [unwired: 7 in, 2 out]
        "RF Linear Velocity (rot/s)" <- w514
        n276 = call "Encoder-Velocity_Conversion (SubVI).vi"("delta  Encoder Count"=w521, "dt (uSec)"=w516) -> ("Rotational Velocity (RPS)"=w511:dbl)  [unwired: 7 in, 2 out]
        "LM Rot Velocity (rot/s)" <- w511
        n277 = call "Encoder-Velocity_Conversion (SubVI).vi"("delta  Encoder Count"=w520, "dt (uSec)"=w516) -> ("Rotational Velocity (RPS)"=w510:dbl)  [unwired: 7 in, 2 out]
        "LF Rot Velocity (rot/s)" <- w510
        n278 = call "Encoder-Velocity_Conversion (SubVI).vi"("delta  Encoder Count"=w519, "dt (uSec)"=w516) -> ("Rotational Velocity (RPS)"=w509:dbl)  [unwired: 7 in, 2 out]
        "RR Rot Velocity (rot/s)" <- w509
        n279 = call "Encoder-Velocity_Conversion (SubVI).vi"("delta  Encoder Count"=w518, "dt (uSec)"=w516) -> ("Rotational Velocity (RPS)"=w513:dbl)  [unwired: 7 in, 2 out]
        "RM Linear Velocity (rot/s)" <- w513
        n280 = Bundle("Rotational Velocity (RPS)"=w512, "Rotational Velocity (RPS)"=w511, "Rotational Velocity (RPS)"=w510, "Rotational Velocity (RPS)"=w509, "Rotational Velocity (RPS)"=w513, "Rotational Velocity (RPS)"=w514) -> (→"Current Rot Velocity (rot/s)":T4)  [unwired: 1 in]
      }
    }
  }
